vi "I2C_Com.vi"() -> ()   [LabVIEW 2019]
uses:
  <vilib>/rvi/Emulation/niFpgaGetClockAttributes.vi
  <vilib>/rvi/Emulation/niFpgaSctlEmulationGetInTimedLoop.vi
  <vilib>/rvi/Emulation/niFpgaEmulationReportErrorSimple.vi
  <vilib>/rvi/Emulation/niFpgaCriticalErrorInLSC.vi
panel:
  in  "Address":bool[](array[boolean])
  in  "Stop":bool
  in  "Data":u8[](array[numeric])=[0, 0, 0, 0, 0, 0, 0, 0]
  out "output data":bool[](array[boolean])
  in  "Read / Write":bool
  in  "Min time SCL Low":u32
  in  "Min time SCL High":u32
  in  "Start":bool
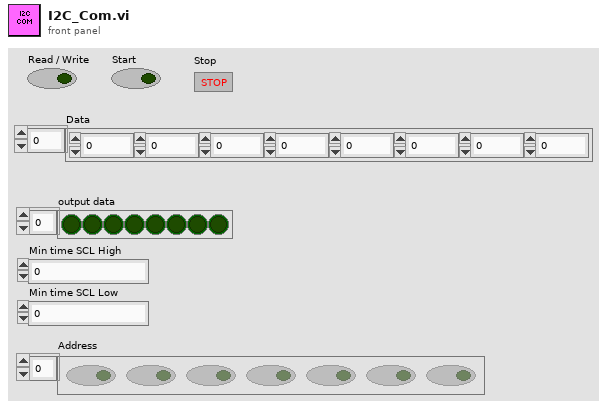
[diagram p1: front panel]
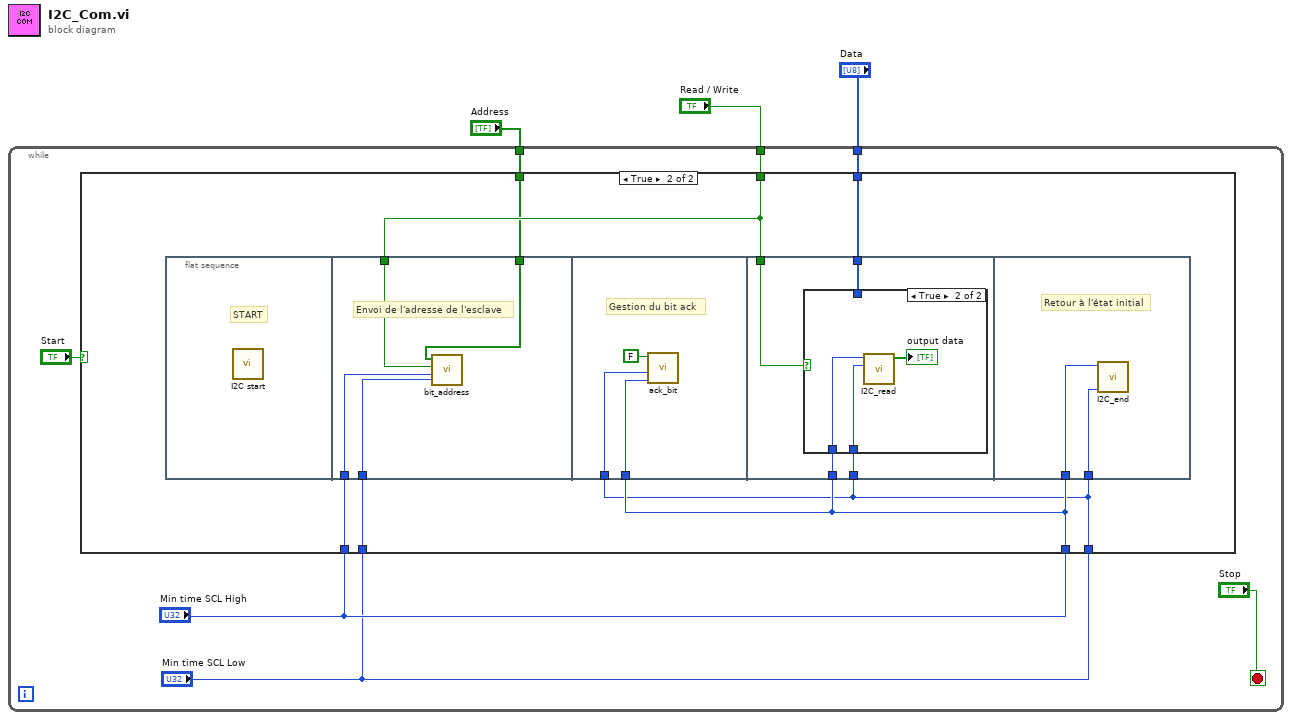
[diagram p0: block diagram]
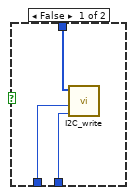
[diagram p3: hidden frame]
diagram:
  n1 = while {
    tunnel: "Read / Write" -> [w7]
    tunnel: "Data" -> [w6]
    tunnel: "Address" -> [w4]
    stop <- "Stop" stop-if-true
    n2 = case shown="True" "Start" {
      tunnel: "Min time SCL High" -> [_ w17]
      tunnel: "Min time SCL Low" -> [_ w16]
      tunnel: "Min time SCL High" -> [_ w14]
      tunnel: "Min time SCL Low" -> [_ w11]
      tunnel: w7 -> [_ w15]
      tunnel: w6 -> [_ w13]
      tunnel: w4 -> [_ w12]
      frame False {
      }
      frame True {
        n3 = flat-sequence {
          tunnel: w17 -> [w21]
          tunnel: w16 -> [w20]
          tunnel: w15 -> [w19]
          tunnel: w12 -> [w18]
          tunnel: w14 -> [w22]
          tunnel: w11 -> [w23]
          tunnel: w15 -> [w28]
          tunnel: w14 -> [w27]
          tunnel: w11 -> [w26]
          tunnel: w13 -> [w25]
          tunnel: w14 -> [w36]
          tunnel: w11 -> [w35]
          frame #0 {
            # "START"
            n4 = call "I2C start.vi"() -> ()  [unwired: 12 in]
          }
          frame #1 {
            # "Envoi de l'adresse de l'esclave"
            n5 = call "bit_address.vi"("Min time SCL Low"=w20, "Min time SCL High"=w21, "Read / Write"=w19, "Address"=w18) -> ()  [unwired: 8 in]
          }
          frame #2 {
            # "Gestion du bit ack"
            n6 = call "ack_bit.vi"("Min time SCL Low"=w22, "Min Time SCL High"=w23, "ack"=FALSE) -> ()  [unwired: 9 in]
          }
          frame #3 {
            n7 = case shown="True" w28 {
              tunnel: w27 -> [w31 w34]
              tunnel: w26 -> [w30 w33]
              tunnel: w25 -> [w29 _]
              frame False {
                n8 = call "I2C_write.vi"("Min time SCL Low"=w30, "Min time SCL High"=w31, "Data"=w29) -> ()  [unwired: 9 in]
              }
              frame True {
                n9 = call "I2C_read.vi"("Min time SCL Low"=w33, "Min Time SCL High"=w34) -> ("reversed array"=→"output data":bool[])  [unwired: 9 in]
              }
            }
          }
          frame #4 {
            # "Retour à l'état initial"
            n10 = call "I2C_end.vi"("Min time SCL Low"=w35, "Min time SCL High"=w36) -> ()  [unwired: 10 in]
          }
        }
      }
    }
  }
